vi "Collect & Clear Error.vi"(8 "Error In":errorcluster) -> (0 "Error Out":errorcluster)   [LabVIEW 2019]
uses:
  Appplicaiton Enviroment/SubVI/Get Development Mode.vi
  User Interface Logger/SubVI/Data Types/Log String.vi
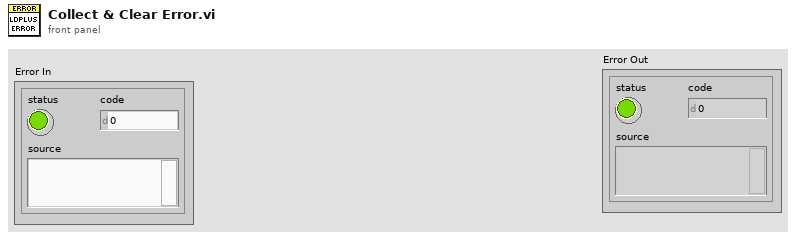
[diagram p1: front panel]
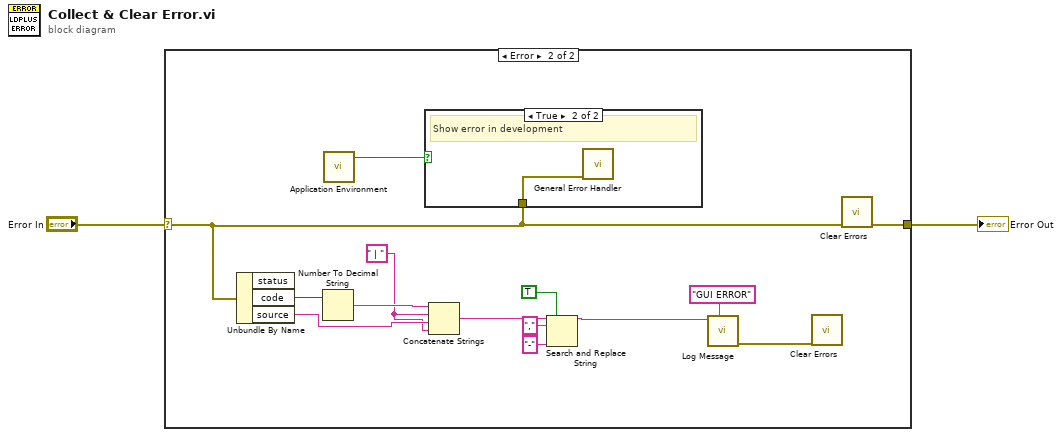
[diagram p0: block diagram]
diagram:
  n1 = case shown="Error" "Error In" {
    selector: "Error In" -> [w3 w12]
    tunnel: [w3 w17] -> w1
    frame No Error {
    }
    frame Error {
      w10 = " | " ("string")
      n2 = Unbundle By Name(w12) -> ("code"=w15:i32, "source"=w13:string)  [unwired: 1 out]
      n3 = Number To Decimal String(number=w15) -> (decimal integer string=w14:string)  [unwired: 1 in]
      n4 = call-poly "Application Environment.vi"() -> ("Development"=w11:bool)  [unwired: 10 in, 1 out]
      n5 = case shown="True" w11 {
        tunnel: w12 -> [_ w18]
        frame False {
        }
        frame True {
          # "Show error in development"
          n6 = call <vilib>:"General Error Handler.vi"("error in (no error)"=w18) -> ()  [unwired: 10 in, 5 out]
        }
      }
      n7 = Concatenate Strings(w14, w10, w13, w10) -> (w9:string)
      n8 = Search and Replace String(replace all?=TRUE ("replace all? (F)"), input string=w9, search string=",", replace string="-" ("replace string (\"\")")) -> (result string=w8:string)  [unwired: 4 in, 3 out]
      n9 = call-poly "Log Message.vi"("Action"="GUI ERROR", "Data"=w8) -> ("Error Out"=w4:errorcluster)  [unwired: 9 in]
      n10 = call <vilib>:"Clear Errors.vi"("error in (no error)"=w4) -> ()  [unwired: 5 in, 2 out]
      n11 = call <vilib>:"Clear Errors.vi"("error in (no error)"=w12) -> ("error out"=w17:errorcluster)  [unwired: 5 in, 1 out]
    }
  }
  "Error Out" <- w1
